vi "Push Sync Files to WebDAV.vi"(0 "AKLH Sync Base":path, 5 "WebDAV IP":string="10.31.176.36", 7 "Sync Time (min)":u32, 9 "WebDAV Push":bool) -> ()   [LabVIEW 2013]
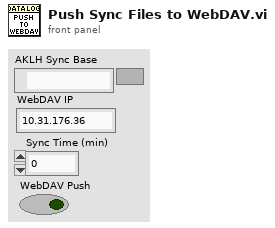
[diagram p1: front panel]
types:
  T1 = typedef "LVDateTimeRec.ctl" = cluster{"fractional second":dbl, "second":i32, "minute":i32, "hour":i32, "day of month":i32, "month":i32, "year":i32, "day of week":i32, "day of year":i32, "DST":i32}
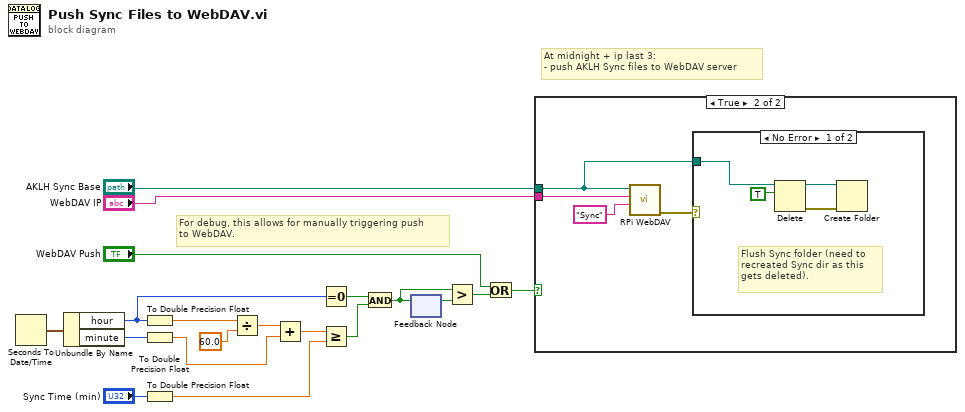
[diagram p0: block diagram]
diagram:
  # "For debug, this allows for manually triggering push\nto WebDAV."
  # "At midnight + ip last 3:\n- push AKLH Sync files to WebDAV server"
  n1 = Seconds To Date/Time() -> (date time rec=w17:T1)  [unwired: 2 in]
  n2 = Unbundle By Name(w17) -> ("hour"=w8:i32, "minute"=w14:i32)
  n3 = To Double Precision Float(number=w8) -> (double precision float=w16:dbl)
  n4 = To Double Precision Float(number=w14) -> (double precision float=w12:dbl)
  n5 = To Double Precision Float(number="Sync Time (min)") -> (double precision float=w9:dbl)
  n6 = Divide(x=w16, y=60.0) -> (x/y=w13:dbl)
  n7 = Add(x=w13, y=w12) -> (x+y=w10:dbl)
  n8 = Equal To 0?(x=w8) -> (x = 0?=w7:bool)
  n9 = Greater Or Equal?(x=w10, y=w9) -> (x >= y?=w6:bool)
  n10 = And(x=w7, y=w6) -> (x .and. y?=w5:bool)
  n11 = feedback-in #1(w5) -> ()
  n12 = feedback #1() -> (w4:bool)  [unwired: 1 in]
  n13 = Greater?(x=w5, y=w4) -> (0:w3:bool)
  n14 = Or(x="WebDAV Push", y=w3) -> (x .or. y?=w1:bool)
  n15 = case shown="True" w1 {
    tunnel: "AKLH Sync Base" -> [_ w20]
    tunnel: "WebDAV IP" -> [_ w23]
    frame False {
    }
    frame True {
      n16 = call "RPi WebDAV.vi"("RPi Sub-Dir"="Sync", "RPi IP"=w23, "RIO Folder"=w20) -> ("Error OUT"=w21:errorcluster)  [unwired: 8 in]
      n17 = case shown="No Error" w21 {
        tunnel: w20 -> [w27 _]
        frame No Error {
          # "Flush Sync folder (need to \nrecreated Sync dir as this\ngets deleted)."
          n18 = Delete(path (use dialog)=w27, entire hierarchy (F)=TRUE ("confirm (F)")) -> (deleted path=w25:path, error out=w24:errorcluster)  [unwired: 3 in, 1 out]
          n19 = Create Folder(path (use dialog)=w25, error in=w24) -> ()  [unwired: 1 in, 3 out]
        }
        frame Error {
          # "If error communicating with\nWebDAV, then leave the files\nalone and try tomorrow."
        }
      }
    }
  }
